vi "EEG_acquisition.vi"() -> ()   [LabVIEW 2020]
uses:
  <vilib>/Analysis/1siggen.llb/Ramp Pattern by Samples.vi
  <vilib>/Analysis/4window.llb/Hamming Window (DBL).vi
  <vilib>/Analysis/2dsp.llb/Real FFT.vi
  <vilib>/Analysis/4window.llb/AllCosWindow (DBL).vi
  <vilib>/Analysis/NI_AALPro.lvlib
  <vilib>/Analysis/NI_AALBase.lvlib
panel:
  in  "Gamma high range":dbl
  in  "Gamma low range":dbl
  out "Gamma Spectrum":cluster{"X":dbl, "Y":dbl}[](graph)
  out "Beta Spectrum":cluster{"X":dbl, "Y":dbl}[](graph)
  in  "Beta high range":dbl
  in  "Beta low range":dbl
  out "Alpha Spectrum":cluster{"X":dbl, "Y":dbl}[](graph)
  out "Frequency resolution":dbl
  in  "Alpha high range":dbl
  in  "Alpha low range":dbl
  out "FFT Spectrum":cluster{dbl, dbl}[](graph)
  in  "Press to stop the script":bool
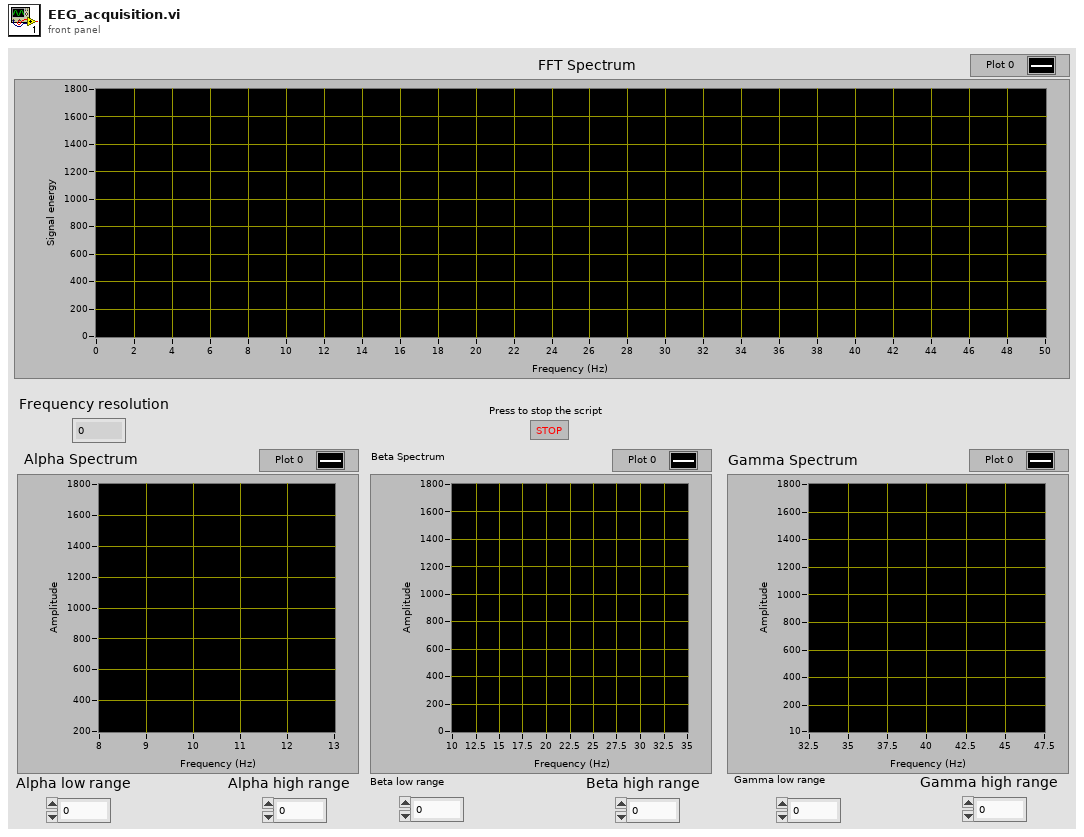
[diagram p1: front panel]
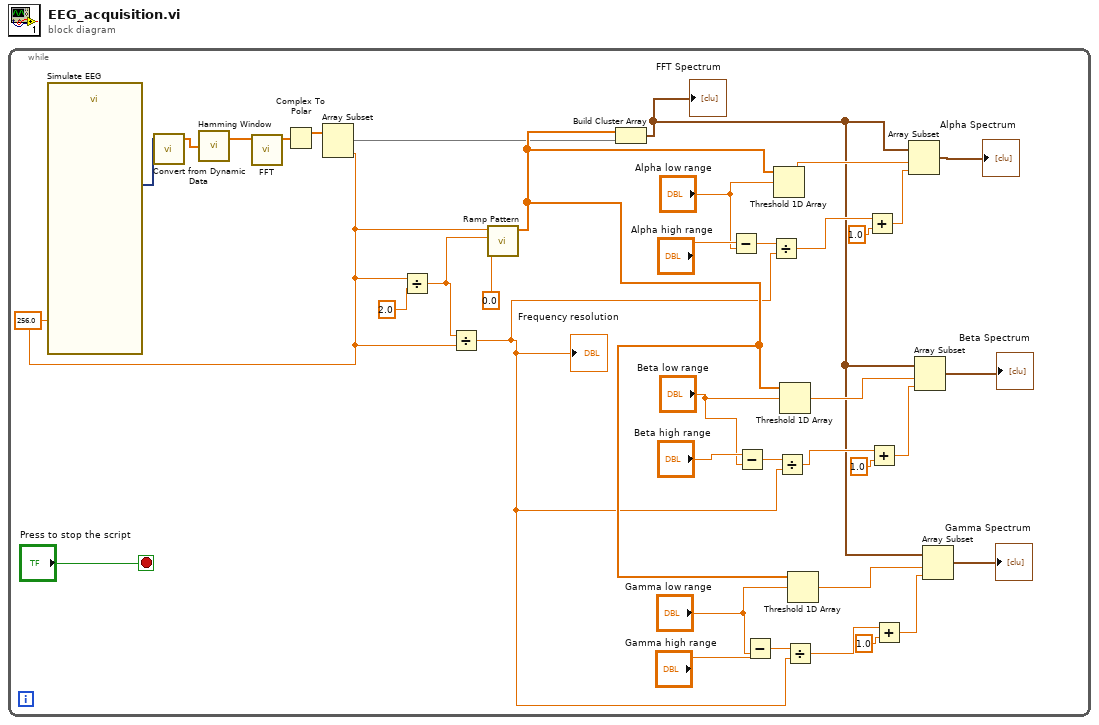
[diagram p0: block diagram]
diagram:
  n1 = while {
    stop <- "Press to stop the script" stop-if-true
    w16 = 256.0 ("sampling rate")
    n2 = call "Simulate EEG"("sampling rate"=w16) -> ("EEG"=w37:dynamicdata)  [unwired: 9 in, 1 out]
    n3 = call "Convert from Dynamic Data"("Dynamic Data Type"=w37) -> ("Array"=w4:dbl[])  [unwired: 3 in]
    n4 = call-poly <vilib>:"Hamming Window.vi"("X"=w4) -> ("Windowed X"=w5:dbl[])  [unwired: 1 out]
    n5 = call-poly <vilib>:"FFT.vi"("X"=w5) -> ("FFT {X}"=w36:cdb[])  [unwired: 9 in, 1 out]
    n6 = Complex To Polar(r * e^(i*theta)=w36) -> (r=w33:dbl[])  [unwired: 1 out]
    n7 = Array Subset(array=w33, length=w16) -> (w3:dbl[])  [unwired: 1 in]
    n8 = Divide(x=w16, y=2.0) -> (x/y=w29:dbl)
    n9 = Divide(x=w29, y=w16) -> (x/y=w15:dbl)
    "Frequency resolution" <- w15
    n10 = call-poly <vilib>:"Ramp Pattern.vi"("start"=0.0, "end"=w29, "samples"=w16) -> ("Ramp Pattern"=w18:dbl[])  [unwired: 7 in, 1 out]
    n11 = Build Cluster Array(w18, w3) -> (w2:cluster{dbl, dbl}[])
    "FFT Spectrum" <- w2
    n12 = Subtract(x="Alpha high range", y="Alpha low range") -> (x-y=w28:dbl)
    n13 = Subtract(x="Beta high range", y="Beta low range") -> (x-y=w25:dbl)
    n14 = Subtract(x="Gamma high range", y="Gamma low range") -> (x-y=w20:dbl)
    n15 = Divide(x=w28, y=w15) -> (x/y=w6:dbl)
    n16 = Threshold 1D Array(2:"Alpha low range", 3:w18) -> (0:w32:dbl)  [unwired: 1 in]
    n17 = Divide(x=w25, y=w15) -> (x/y=w10:dbl)
    n18 = Threshold 1D Array(2:"Beta low range", 3:w18) -> (0:w24:dbl)  [unwired: 1 in]
    n19 = Divide(x=w20, y=w15) -> (x/y=w14:dbl)
    n20 = Threshold 1D Array(2:"Gamma low range", 3:w18) -> (0:w19:dbl)  [unwired: 1 in]
    n21 = Add(x=w6, y=1.0) -> (x+y=w7:dbl)
    n22 = Add(x=w10, y=1.0) -> (x+y=w9:dbl)
    n23 = Add(x=w14, y=1.0) -> (x+y=w13:dbl)
    n24 = Array Subset(array=w2, index=w32, length=w7) -> (→"Alpha Spectrum":cluster{dbl, dbl}[])
    n25 = Array Subset(array=w2, index=w24, length=w9) -> (→"Beta Spectrum":cluster{dbl, dbl}[])
    n26 = Array Subset(array=w2, index=w19, length=w13) -> (→"Gamma Spectrum":cluster{dbl, dbl}[])
  }
